vi "CheckPauseBetweenTimeString.vi"(8 "greater than (s)":dbl=60.0, 10 "laterEntry":string[](array[string])=["15:54", "902_3218_call1", "3", "2,5", "3"], 11 "earlierEntry":string[](array[string])=["15:53", "902_3218_call1", "3", "2,5", "3"]) -> (0 "pause ok":bool, 3 "pause":dbl=60.0)   [LabVIEW 2014]
panel:
  out "output 2":timestamp=timestamp(53580 s since 1904-01-01)
  out "output 1":timestamp=timestamp(53640 s since 1904-01-01)
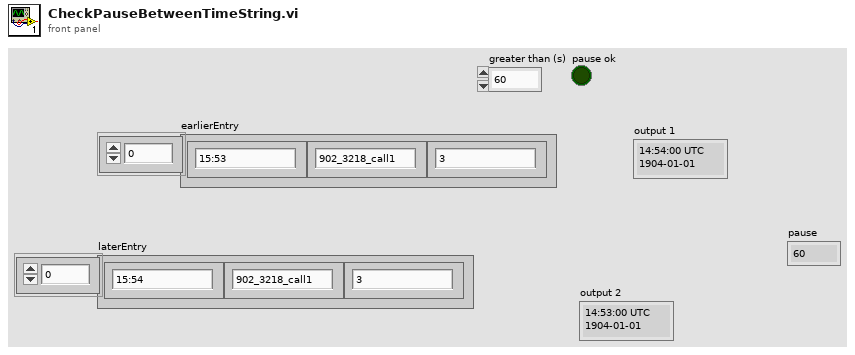
[diagram p1: front panel]
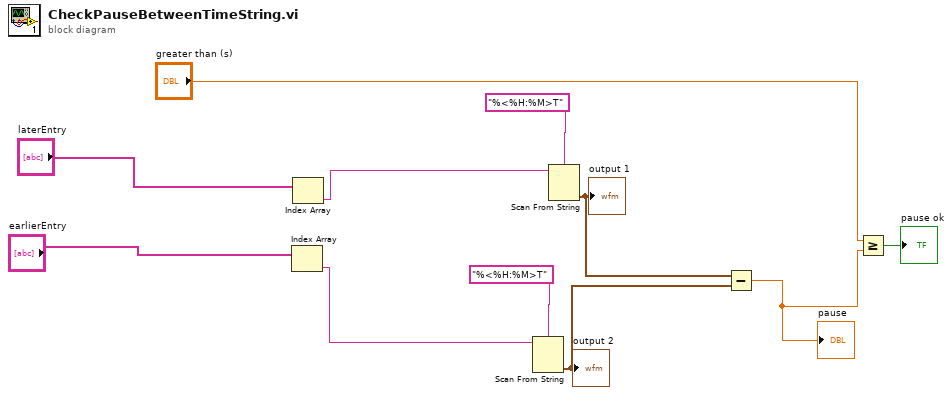
[diagram p0: block diagram]
diagram:
  n1 = Index Array(array="earlierEntry") -> (element=w8:string)  [unwired: 1 in]
  n2 = Index Array(array="laterEntry") -> (element=w10:string)  [unwired: 1 in]
  n3 = Scan From String(format string="%<%H:%M>T", input string=w8) -> (output 1=w4:timestamp)  [unwired: 3 in, 3 out]
  "output 2" <- w4
  n4 = Scan From String(format string="%<%H:%M>T", input string=w10) -> (output 1=w5:timestamp)  [unwired: 3 in, 3 out]
  "output 1" <- w5
  n5 = Subtract(x=w5, y=w4) -> (x-y=w2:dbl)
  "pause" <- w2
  n6 = Greater Or Equal?(x="greater than (s)", y=w2) -> (x >= y?=→"pause ok":bool)
